vi "Actor Core.vi"(8 "error in":errorcluster, 11 "Elevator Controller in":refnum<class "Elevator Controller Actor.lvclass">) -> (0 "error out":errorcluster, 3 "Actor out":refnum<class "Actor.lvclass">)   [LabVIEW 2019, in "Elevator Controller Actor.lvlib" / "Elevator Controller Actor.lvclass"]
doc: "(<B>Filename</B>: Actor Framework.lvlib:Actor.lvclass:Actor Core.vi)\n\nReceives messages to the actor, reacts to them, and initiates any error handling that may shut the actor down.\n\nDescendant classes may override this VI to append parallel tasks for the actor to complete while it handles messages. Overrides use the Call Parent Method node."
uses:
  Elevator Controller Actor.lvclass
  <vilib>/ActorFramework/Stop Msg/Stop Msg.lvclass
  <vilib>/ActorFramework/Actor/Actor.lvclass
  C:/Program Files (x86)/National Instruments/LabVIEW 2019/vi.lib/ActorFramework/Actor/Actor.lvclass
panel:
  # "Elevator Controller"
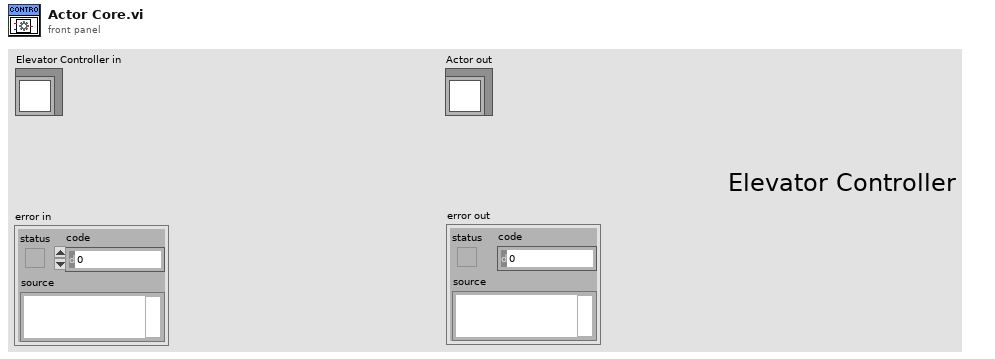
[diagram p1: front panel]
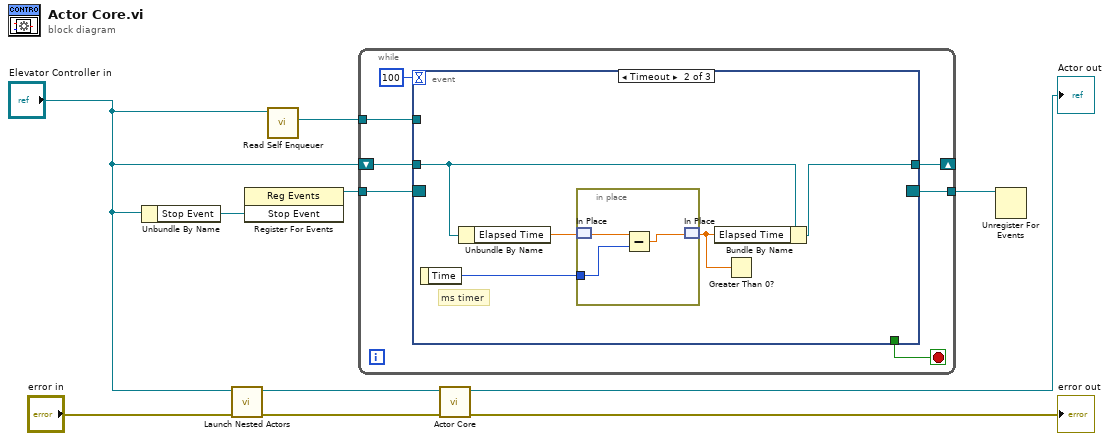
[diagram p0: block diagram]
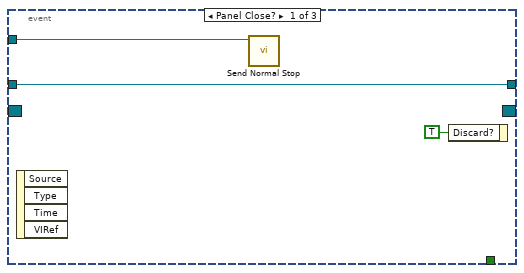
[diagram p2: hidden frame]
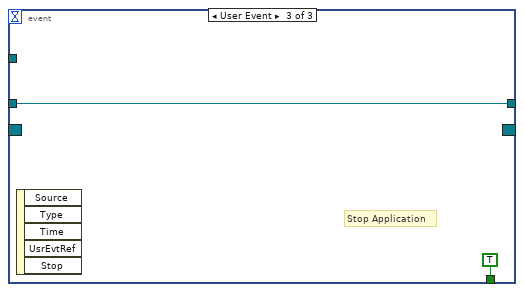
[diagram p3: hidden frame]
diagram:
  n1 = Unbundle By Name("Elevator Controller in") -> ("Stop Event"=w8:refnum<user-event>)
  n2 = call "Launch Nested Actors.vi"("error in (no error)"="error in", "Elevator Controller Actor in"="Elevator Controller in") -> ("error out"=w3:errorcluster, "Elevator Controller Actor out"=w2:refnum<class "Elevator Controller Actor.lvclass">)  [unwired: 8 in]
  n3 = register-events(w8) -> (reference out=w7:refnum<event-registration>)  [unwired: 2 in, 1 out]
  n4 = call <vilib>:"Read Self Enqueuer.vi"("Actor"="Elevator Controller in") -> ("Self Enqueuer"=w5:refnum<class "Message Enqueuer.lvclass">)  [unwired: 10 in]
  n5 = while {
    tunnel: w7 -> [w16]
    tunnel: [w15] -> w6
    tunnel: w5 -> [w14]
    shift-right: [w11] -> _
    shift-left: "Elevator Controller in" -> [w12]
    stop <- w17 stop-if-true
    n6 = event shown="[1] Timeout" {
      selector: w16 -> [_ _ _]
      dyn-events: [_ _ _] -> w15
      timeout: 100 -> [_ _ _]
      tunnel: [_ _ TRUE] -> w17
      tunnel: w14 -> [w19 _ _]
      tunnel: w12 -> [w18 w25 w29]
      tunnel: [w18 w24 w29] -> w11
      event Panel Close? {
        n7 = event-data() -> ()  [unwired: 1 in, 4 out]
        n8 = call <vilib>:"Send Normal Stop.vi"("Message Enqueuer"=w19) -> ()  [unwired: 10 in, 1 out]
        n9 = event-data("Discard?"=TRUE) -> ()  [unwired: 1 in, 1 out]
      }
      event Timeout {
        # "ms timer"
        n10 = event-data() -> ("Time"=w23:u32)  [unwired: 1 in]
        n11 = Unbundle By Name(w25) -> ("Elapsed Time"=w22:dbl)
        n12 = in-place {
          in-place-border: w23 -> [w27]
          n13 = in-place-match #1(w22) -> (w28:dbl)
          n14 = Subtract(x=w28, y=w27) -> (x-y=w26:dbl)
          n15 = in-place-match #1(w26) -> (w21:dbl)
        }
        n16 = Bundle By Name(cluster=w25, "Elapsed Time"=w21) -> (w24:refnum<class "Elevator Controller Actor.lvclass">)
        n17 = Greater Than 0?(x=w21) -> ()  [unwired: 1 out]
      }
      event User Event {
        # "Stop Application"
        n18 = event-data() -> ()  [unwired: 1 in, 5 out]
      }
    }
  }
  n19 = call-parent "Actor Core.vi"("error in"=w3, "Actor in"=w2) -> ("error out"=→"error out":errorcluster, "Actor out"=→"Actor out":refnum<class "Actor.lvclass">)  [unwired: 8 in]
  n20 = Unregister For Events(event registration refnum=w6) -> ()  [unwired: 1 in, 1 out]
